vi "Auto Auger SM.vi"(9 "Frisbees In":i8, 10 "Index Down":bool, 11 "Index Up":bool) -> (1 "Number of Frisbees Out":i8, 2 "Setpoint Out":dbl)   [LabVIEW 2012]
uses:
  typedefs/subStates.ctl
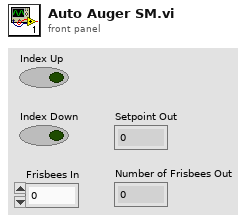
[diagram p1: front panel]
types:
  T1 = typedef "subStates.ctl" = enum16{"null", "wait", "driver control", "auto", "manual override", "hold position", "rotate", "feeder", "end"}
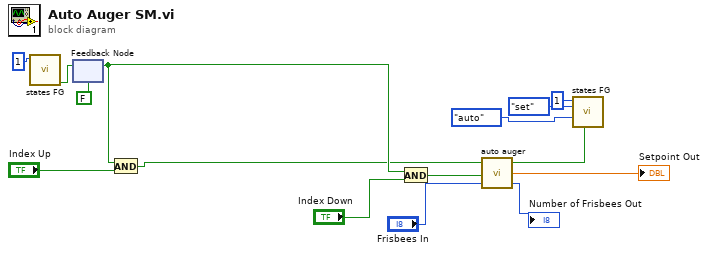
[diagram p0: block diagram]
diagram:
  n1 = call "states FG.vi"("Loop ID"=1) -> ("first call?"=w3:bool)  [unwired: 7 in, 3 out]
  n2 = feedback #1(FALSE) -> (w2:bool)
  n3 = feedback-in #1(w3) -> ()
  n4 = And(x=w2, y="Index Up") -> (x .and. y?=w1:bool)
  n5 = And(x=w2, y="Index Down") -> (x .and. y?=w14:bool)
  n6 = call "auto auger.vi"("Number of Frisbees"="Frisbees In", "Index Down"=w14, "Index Up"=w1) -> ("Number of Frisbees Out"=→"Number of Frisbees Out":i8, "Setpoint Out"=→"Setpoint Out":dbl, "Finished"=w9:bool)
  n7 = call "states FG.vi"("exit in"=w9, "subState in"=subStates."auto", "menu (get)"=enum16{"set", "get"}."set", "Loop ID"=1) -> ()  [unwired: 4 in, 4 out]
